vi "Quick Start - Write Custom Cluster.vi"() -> ()   [LabVIEW 2020]
uses:
  Nominal Client/Nominal Client.lvclass/Nominal Client.ctl
  68d6fcb1-550e-49ab-bce3-21796ae30af0.vi
  Nominal Client/http.post.vi
  Nominal Client/private_data.set.vi
  68d6fcb1-550e-49ab-bce3-21796ae30af0.vi/8284acbc-2d4d-4b18-b492-8ff51a6e7e10.vi
  Nominal Client/trace.payload_received.vi
  Nominal Client/error.vi
  Nominal Client/trace.payload_sent.vi
  Nominal Client/create.authorization_header.vi
  nominal types/workspace/id.get.vi
  nominal types/workspace/rid.get.vi
  <vilib>/AdvancedString/1D String Array to Delimited String.vi
  Nominal Client/workspace.set.vi
  Nominal Client/trace.calling_method.vi
  Nominal Client/error.vi/859f8e04-e495-489b-b5b4-7ac163f56130.vi
  <vilib>/JDP Science/JDP Science Common Utilities/Trim Whitespace__JDP.vi
  Nominal Client/api_token.get.vi
  <vilib>/Utility/file.llb/Application Directory.vi
  <vilib>/Utility/error.llb/Error Cluster From Error Code.vi
  Nominal Client/format endpoint termination.vi
  submodules/reqwest-labview/lv-src/reqwest/create.vi
  Nominal Client/workspace_cache.get_from_rid.vi
  Nominal Client/workspace_cache.get.vi
  Nominal Client/Palette Items/who_am_i.vi
  stream_custom_cluster/to json.vi
  <vilib>/Utility/libraryn.llb/Get File Extension.vi
  Nominal Client/log_file.write.vi
  submodules/reqwest-labview/lv-src/reqwest/post.vi
  <vilib>/JDP Science/JSONtext/Get all Object Items.vi
  <vilib>/JDP Science/JSONtext/JSON text to Variant.vi
  User/User.lvclass
  Nominal Client/Nominal Client.lvclass
  nominal types/workspace/workspace.lvclass
  submodules/reqwest-labview/lv-src/reqwest/reqwest.lvclass
  <vilib>/JDP Science/JSONtext/LVClass Serializer/JSONtext LVClass Serializer.lvclass
  stream_custom_cluster/stream_custom_cluster.lvclass
panel:
  in  "API Token (string or path)":string
  in  "Data Source RID":string
  out "Consumer Stopped":bool
  in  "Data Cluster":T1 {"asdfHorizontal Pointer Slide" scale=0.0..10.0}
  in  "Stop":bool
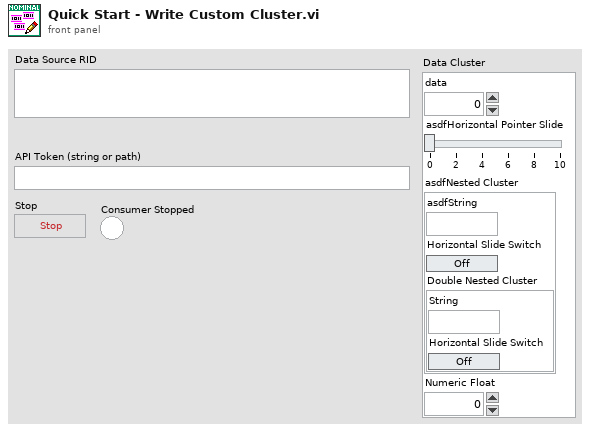
[diagram p1: front panel]
types:
  T1 = cluster{"data":i32, "asdfHorizontal Pointer Slide":dbl, "asdfNested Cluster":cluster{"asdfString":string, "Horizontal Slide Switch":bool, "Double Nested Cluster":cluster{"String":string, "Horizontal Slide Switch":bool}}, "Numeric Float":dbl}
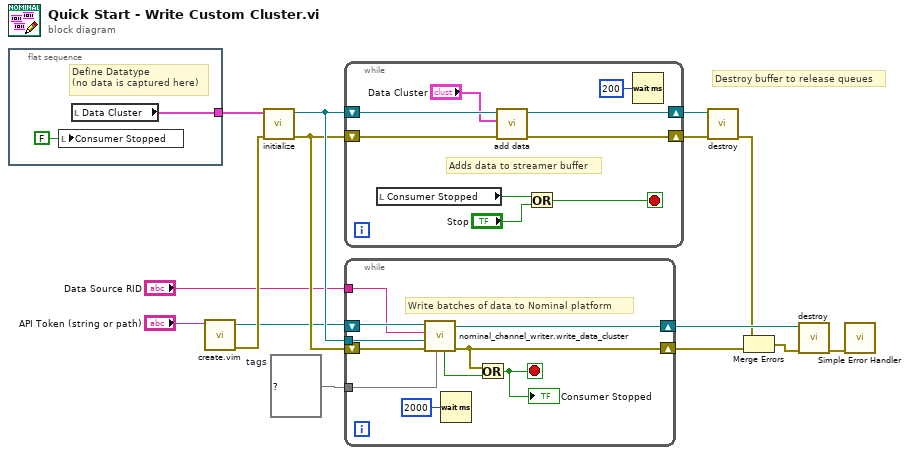
[diagram p0: block diagram]
diagram:
  w1 = map{string, string} {}  # tags
  # "Destroy buffer to release queues"
  n1 = flat-sequence {
    tunnel: [w17] -> w11
    frame #0 {
      # "Define Datatype\n(no data is captured here)"
      n2 = local write "Consumer Stopped"(FALSE ("Consumer Stopped")) -> ()
      n3 = local read "Data Cluster"() -> (w17:T1)
    }
  }
  n4 = call "create.vim"("API Token (string or path)"="API Token (string or path)") -> ("error out"=w10:errorcluster, "Nominal Client"=w2:refnum<class "Nominal Client.lvclass">)  [unwired: 8 in, 1 out]
  n5 = call "initialize.vi"("error in"=w10, "Data Cluster"=w11) -> ("error out"=w13:errorcluster, "stream custom cluster"=w14:refnum<class "stream_custom_cluster.lvclass">)  [unwired: 8 in]
  n6 = while {
    shift-right: [w22] -> w12
    shift-left: w13 -> [w23]
    shift-right: [w25] -> w15
    shift-left: w14 -> [w26]
    stop <- w18 stop-if-true
    # "Adds data to streamer buffer"
    n7 = local read "Consumer Stopped"() -> (w20:bool)
    n8 = call "add data.vi"("error in"=w23, "Data Cluster"="Data Cluster", "stream custom cluster in"=w26) -> ("error out"=w22:errorcluster, "stream custom cluster out"=w25:refnum<class "stream_custom_cluster.lvclass">)  [unwired: 7 in]
    n9 = Or(x=w20, y="Stop") -> (x .or. y?=w18:bool)
    n10 = Wait (ms)(milliseconds to wait=u32 200) -> ()  [unwired: 1 out]
  }
  n11 = while {
    tunnel: w14 -> [w35]
    shift-right: [w32] -> w9
    shift-left: w2 -> [w33]
    tunnel: "Data Source RID" -> [w31]
    shift-right: [w30] -> w5
    shift-left: w13 -> [w34]
    tunnel: w1 -> [w27]
    stop <- w28 stop-if-true
    # "Write batches of data to Nominal platform"
    n12 = call "nominal_channel_writer.write_data_cluster.vi"("tags"=w27, "error in"=w34, "Custom Cluster Streamer"=w35, "Data Source RID"=w31, "Nominal Client in"=w33) -> ("error out"=w30:errorcluster, "Nominal Client out"=w32:refnum<class "Nominal Client.lvclass">, "Terminated"=w29:bool)  [unwired: 4 in]
    n13 = Wait (ms)(milliseconds to wait=u32 2000) -> ()  [unwired: 1 out]
    n14 = Or(x=w30, y=w29) -> (x .or. y?=w28:bool)
    "Consumer Stopped" <- w28
  }
  n15 = call "destroy.vi"("error in"=w12, "stream custom cluster"=w15) -> ("error out"=w6:errorcluster)  [unwired: 9 in]
  n16 = Merge Errors(w6, w5) -> (w4:errorcluster)
  n17 = call "destroy.vi"("error in"=w4, "Nominal Client"=w9) -> ("error out"=w3:errorcluster)  [unwired: 9 in]
  n18 = call <vilib>:"Simple Error Handler.vi"("error in (no error)"=w3) -> ()  [unwired: 4 in, 5 out]
